vi "GetEnumValue.vi"(8 "error in (no error)":errorcluster caption="错误输入（无错误）", 10 "strKey":string, 11 "handle":u64) -> (0 "error out":errorcluster caption="错误输出", 1 "pEnumValue out":T1, 2 "function return":i32, 3 "handle out":u64)   [LabVIEW 2011, in "MvCameraControl.lvlib"]
doc: "MV_LV_API int __stdcall GetEnumValue( void* handle, const char* strValue, MVCC_ENUMVALUE *pEnumValue);"
uses:
  MvCameraControl.lvlib
  MvCameraControl.dll
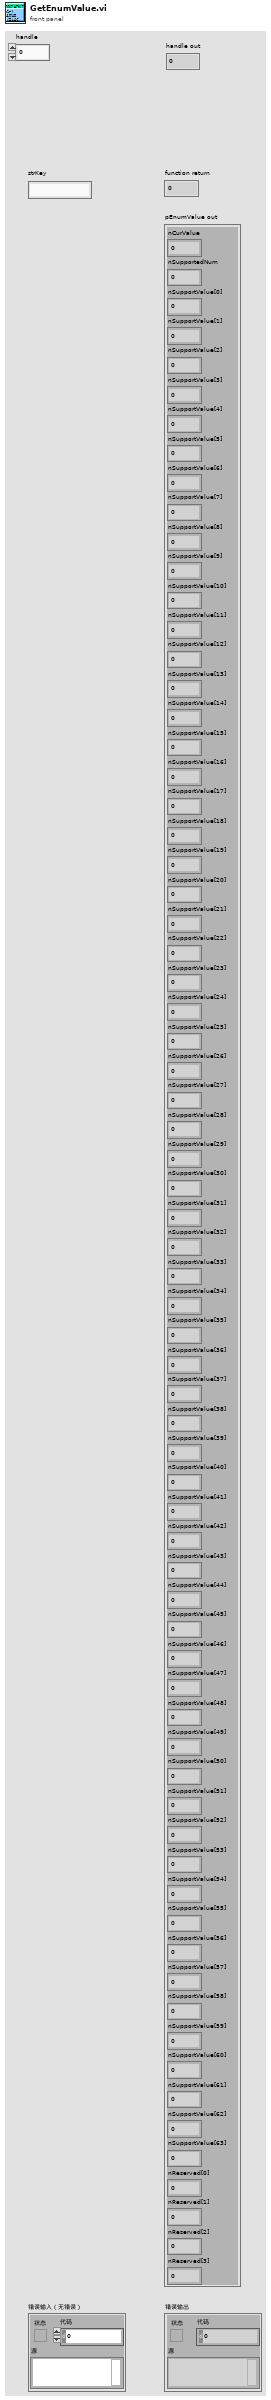
[diagram p1: front panel]
types:
  T1 = cluster{"nCurValue":u32, "nSupportedNum":u32, "nSupportValue[0]":u32, "nSupportValue[1]":u32, "nSupportValue[2]":u32, "nSupportValue[3]":u32, "nSupportValue[4]":u32, "nSupportValue[5]":u32, "nSupportValue[6]":u32, "nSupportValue[7]":u32, "nSupportValue[8]":u32, "nSupportValue[9]":u32, "nSupportValue[10]":u32, "nSupportValue[11]":u32, "nSupportValue[12]":u32, "nSupportValue[13]":u32, "nSupportValue[14]":u32, "nSupportValue[15]":u32, "nSupportValue[16]":u32, "nSupportValue[17]":u32, "nSupportValue[18]":u32, "nSupportValue[19]":u32, "nSupportValue[20]":u32, "nSupportValue[21]":u32, "nSupportValue[22]":u32, "nSupportValue[23]":u32, "nSupportValue[24]":u32, "nSupportValue[25]":u32, "nSupportValue[26]":u32, "nSupportValue[27]":u32, "nSupportValue[28]":u32, "nSupportValue[29]":u32, "nSupportValue[30]":u32, "nSupportValue[31]":u32, "nSupportValue[32]":u32, "nSupportValue[33]":u32, "nSupportValue[34]":u32, "nSupportValue[35]":u32, "nSupportValue[36]":u32, "nSupportValue[37]":u32, "nSupportValue[38]":u32, "nSupportValue[39]":u32, "nSupportValue[40]":u32, "nSupportValue[41]":u32, "nSupportValue[42]":u32, "nSupportValue[43]":u32, "nSupportValue[44]":u32, "nSupportValue[45]":u32, "nSupportValue[46]":u32, "nSupportValue[47]":u32, "nSupportValue[48]":u32, "nSupportValue[49]":u32, "nSupportValue[50]":u32, "nSupportValue[51]":u32, "nSupportValue[52]":u32, "nSupportValue[53]":u32, "nSupportValue[54]":u32, "nSupportValue[55]":u32, "nSupportValue[56]":u32, "nSupportValue[57]":u32, "nSupportValue[58]":u32, "nSupportValue[59]":u32, "nSupportValue[60]":u32, "nSupportValue[61]":u32, "nSupportValue[62]":u32, "nSupportValue[63]":u32, "nReserved[0]":u32, "nReserved[1]":u32, "nReserved[2]":u32, "nReserved[3]":u32}
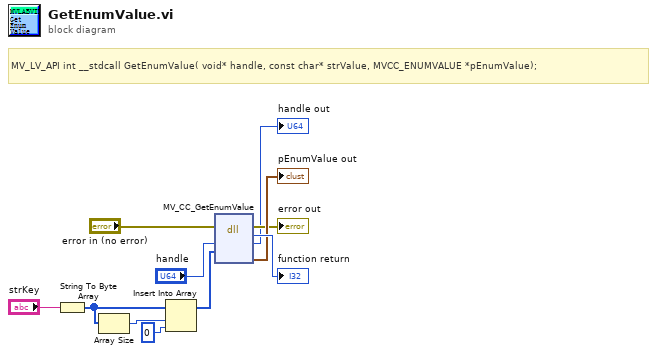
[diagram p0: block diagram]
diagram:
  # "MV_LV_API int __stdcall GetEnumValue( void* handle, const char* strValue, MVCC_ENUMVALUE *pEnumValue);"
  n1 = String To Byte Array(string="strKey") -> (unsigned byte array=w7:u8[])
  n2 = Array Size(array=w7) -> (size(s)=w6:i32)
  n3 = Insert Into Array(array=w7, index=w6, new element=u8 0 ("新元素/子数组")) -> (w3:u8[])
  n4 = dll-call lib="MvCameraControl.dll" fn="MV_CC_GetEnumValue"(error in="error in (no error)", "handle"="handle", "strKey"=w3) -> (error out=→"error out":errorcluster, "返回类型"=→"function return":i32, "handle"=→"handle out":u64, "pEnumValue out"=→"pEnumValue out":T1)  [unwired: 4 in, 1 out]
